vi "ScopeClock.vi"(8 "error in (no error)":errorcluster caption="错误输入（无错误）", 10 "fre(Hz)":i32=800000, 11 "handle":u64) -> (0 "error out":errorcluster caption="错误输出", 2 "function return":i32, 3 "handle out":u64)   [LabVIEW 2018]
doc: "Set Scope AD Clock Frequency \nMax 40MHz ,then div by int as 20MHz 10MHz..."
uses:
  InstrumentsPlayground.lvlib
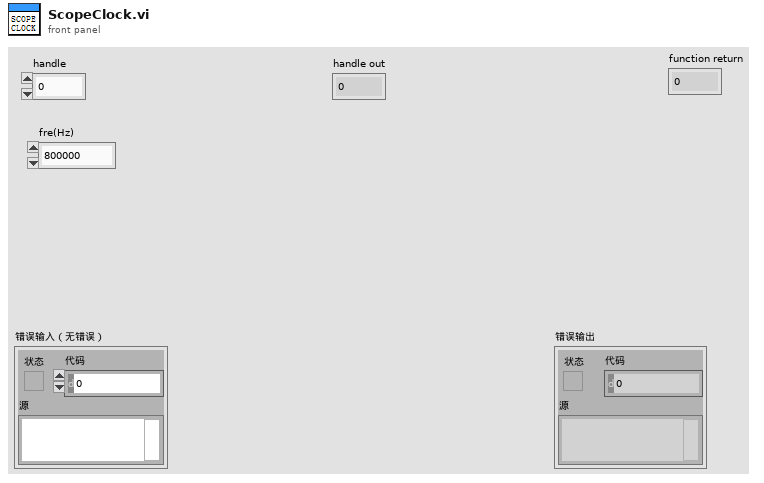
[diagram p1: front panel]
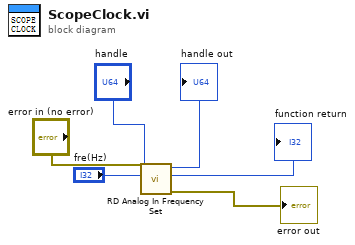
[diagram p0: block diagram]
diagram:
  n1 = call "RD Analog In Frequency Set.vi"("error in (no error)"="error in (no error)", "fre"="fre(Hz)", "handle"="handle") -> ("error out"=→"error out":errorcluster, "function return"=→"function return":i32, "handle out"=→"handle out":u64)  [unwired: 6 in]
